vi "Simple time series player window menu.vi"(8 "error in (no error)":errorcluster, 11 "menu":refnum<k9>) -> (0 "error out":errorcluster, 3 "menu reference out":refnum<k9>)   [LabVIEW 2020]
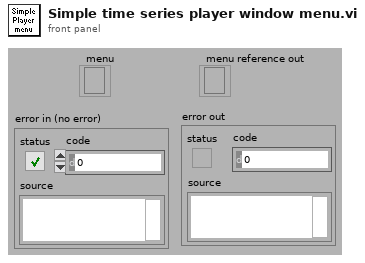
[diagram p1: front panel]
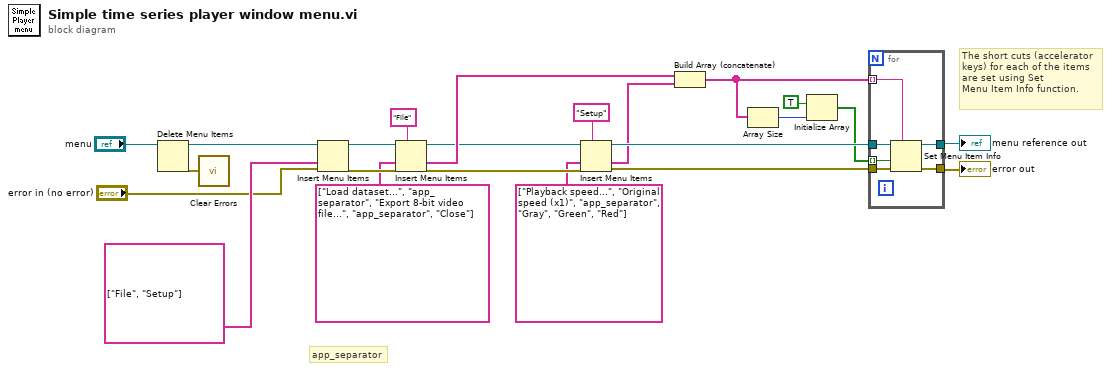
[diagram p0: block diagram]
diagram:
  # "app_separator"
  # "The short cuts (accelerator\nkeys) for each of the items\nare set using Set\nMenu Item Info function."
  n1 = Delete Menu Items(9:"menu") -> (0:w12:errorcluster, 3:w19:refnum<k9>)  [unwired: 2 in, 1 out]
  n2 = call <vilib>:"Clear Errors.vi"("error in (no error)"=w12) -> ()  [unwired: 5 in, 2 out]
  n3 = Insert Menu Items(6:"error in (no error)", 7:string[] ["File", "Setup"] ("item tags"), 9:w19) -> (0:w21:errorcluster, 3:w13:refnum<k9>)  [unwired: 4 out]
  n4 = Insert Menu Items(5:"File" ("menu tag"), 6:w21, 7:string[] ["Load dataset...", "app_separator", "Export 8-bit video file...", "app_separator", "Close"] ("item tags"), 9:w13) -> (0:w22:errorcluster, 1:w18:string[], 3:w14:refnum<k9>)  [unwired: 2 out]
  n5 = Insert Menu Items(5:"Setup" ("menu tag"), 6:w22, 7:string[] ["Playback speed...", "Original speed (x1)", "app_separator", "Gray", "Green", "Red"] ("item tags"), 9:w14) -> (0:w10:errorcluster, 1:w8:string[], 3:w9:refnum<k9>)  [unwired: 2 out]
  n6 = Build Array (concatenate)(w18, w8) -> (w5:string[])
  n7 = Array Size(array=w5) -> (size(s)=w7:i32)
  n8 = Initialize Array(TRUE, w7) -> (w6:bool[])
  n9 = for {
    tunnel: w9 -> [w29]
    tunnel: [w28] -> w16
    tunnel: w5 -> [w27] mode=indexing
    tunnel: w10 -> [w26]
    tunnel: [w25] -> w23
    tunnel: w6 -> [w24] mode=indexing
    n10 = Set Menu Item Info(7:w27, 8:w26, 9:w24, 11:w29) -> (0:w25:errorcluster, 3:w28:refnum<k9>)  [unwired: 1 in, 2 out]
  }
  "error out" <- w23
  "menu reference out" <- w16
